vi "TCL Log Baseline to Disk.vi"(0 "Event":string[](array[string])) -> ()   [LabVIEW 2009]
uses:
  TCL Global.vi
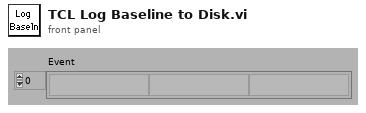
[diagram p1: front panel]
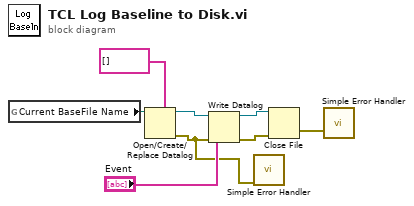
[diagram p0: block diagram]
diagram:
  n1 = global read "TCL Global.vi" "Current BaseFile Name"() -> (w4:path)
  n2 = Open/Create/Replace Datalog(5:string[] [], 11:w4) -> (0:w2:errorcluster, 3:w7:refnum<k1>)  [unwired: 4 in, 1 out]
  n3 = Write Datalog(4:w2, 6:"Event", 7:w7) -> (0:w3:errorcluster, 3:w6:refnum<k1>)
  n4 = call <vilib>:"Simple Error Handler.vi"("error in (no error)"=w2) -> ()  [unwired: 4 in, 5 out]
  n5 = Close File(refnum=w6, error in=w3) -> (error out=w1:errorcluster)  [unwired: 1 out]
  n6 = call <vilib>:"Simple Error Handler.vi"("error in (no error)"=w1) -> ()  [unwired: 4 in, 5 out]
